vi "Actor Core.vi"(8 "error in":errorcluster, 11 "Top Level in":refnum<class "Top Level.lvclass">) -> (0 "error out":errorcluster, 3 "Actor out":refnum<class "Actor.lvclass">)   [LabVIEW 2020, in "2. Basic Panel Actors.lvlib" / "Top Level.lvclass"]
doc: "The user interface for this panel.\n----\nCopyright: MGI 2016\nAuthor: Derek Trepanier"
uses:
  Top Level.lvclass
  C:/Program Files/National Instruments/LabVIEW 2020/vi.lib/MGI/Panel Manager/Panel Actor/Panel Actor/Panel Actor.lvclass
  <vilib>/ActorFramework/Actor/Actor.lvclass
  <vilib>/ActorFramework/Message Enqueuer/Message Enqueuer.lvclass/Message Enqueuer.ctl
  Instrument/DMM/DMM.lvclass
  Instrument/Power Supply/Power Supply.lvclass
  <vilib>/ActorFramework/Message Enqueuer/Enqueue.vi
  Description Panel/Description Panel.lvclass
  <vilib>/MGI/Panel Manager/Panel/Panel/Subpanel/Subpanel.lvclass
  C:/Program Files/National Instruments/LabVIEW 2020/vi.lib/MGI/Panel Manager/Panel/Panel/Panel.lvclass
  <vilib>/ActorFramework/Stop Msg/Stop Msg.lvclass
  C:/Program Files/National Instruments/LabVIEW 2020/vi.lib/ActorFramework/Message/Message.lvclass
  <vilib>/MGI/Panel Manager/Panel/Panel/Window/Window.lvclass
  <vilib>/MGI/Panel Manager/Panel/Panel/Subpanel/Subpanel.vi
  <vilib>/ActorFramework/Message Priority Queue/Priority Enqueue.vi
  <vilib>/MGI/Panel Manager/Panel/Panel/Window/Window.vi
  <vilib>/MGI/Panel Manager/Panel Actor/Panel Actor/Panel Actor.lvclass
  <vilib>/MGI/Panel Manager/Panel/Panel.lvlib
panel:
  in  "Config Power Supply":bool
  in  "Config DMM":bool
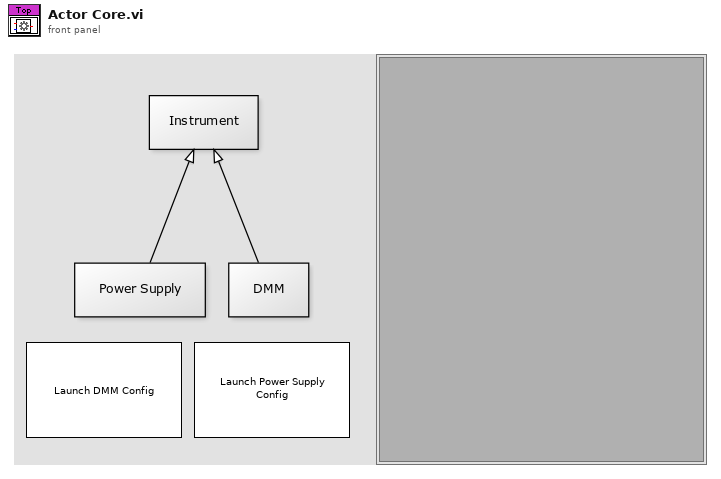
[diagram p1: front panel]
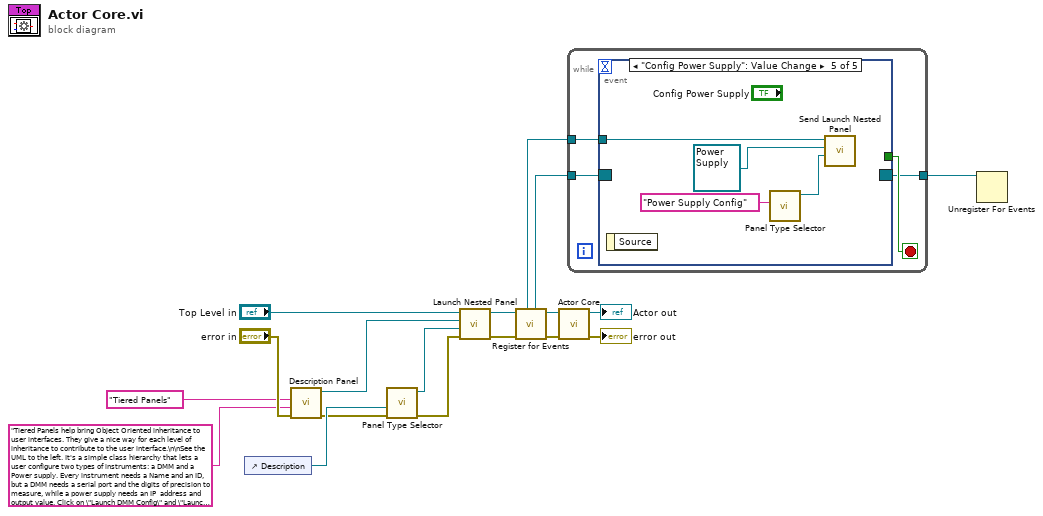
[diagram p0: block diagram]
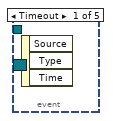
[diagram p2: hidden frame]
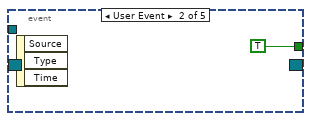
[diagram p3: hidden frame]
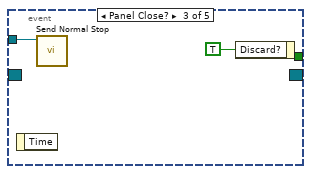
[diagram p4: hidden frame]
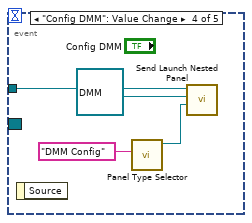
[diagram p5: hidden frame]
diagram:
  n1 = control-ref of="Description"() -> (w8:refnum<vi>)
  n2 = call "Description Panel.vi"("error in (no error)"="error in", "Description"="Tiered Panels help bring Object Oriented inheritance to user interfaces. They give a nice way for each level of inheritance to contribute to the user interface.\n\nSee the UML to the left. It's a simple class hierarchy that lets a user configure two types of instruments: a DMM and a Power supply. Every instrument needs a Name and an ID, but a DMM needs a serial port and the digits of precision to measure, while a power supply needs an IP  address and output value. Click on \"Launch DMM Config\" and \"Launch Power Supply Config\" and compare the two user interfaces. They both have the same \"Name\", \"ID\", and \"Save\" controls, but they have different \"Configuration\" controls.\n\nNow look at the Power Supply Config user interface. It's the Front Panel of \"Power Supply.lvclass:Actor Core.vi\". Notice how it only has the power supply specific controls. Just like how \"DMM.lvclass:Actor Core.vi\" only contains the DMM Specific controls.\n\nFinally, look at the Insturment's user interface in \"Instrument.lvclass:Actor Core.vi\". This contains only controls that are specific to <b>all</b> instruments, like the Name and the ID, as well as a button to save the configuration. It also contains a subpanel. This is where the specific instrument's UI will be inserted. Check out the block diagram of the Instrument's UI to see how to implement this. The bookmark <b>#TieredPanels</b> will explain how to make this work.\n" ("Description Title"), "Description Title"="Tiered Panels") -> ("error out"=w7:errorcluster, "Description Panel out"=w6:refnum<class "Description Panel.lvclass">)  [unwired: 7 in]
  n3 = call-poly <vilib>:"Panel Type Selector.vi"("Error In"=w7, "Sub Panel"=w8) -> ("Error Out"=w9:errorcluster, "Subpanel Out"=w2:refnum<class "Subpanel.lvclass">)  [unwired: 8 in]
  n4 = call <vilib>:"Launch Nested Panel.vi"("error in (no error)"=w9, "Panel"=w2, "Nested Panel Actor"=w6, "Panel Actor in"="Top Level in") -> ("error out"=w12:errorcluster, "Panel Actor out"=w10:refnum<class "Top Level.lvclass">)  [unwired: 4 in, 2 out]
  n5 = call <vilib>:"Register for Events.vi"("Error In"=w12, "Panel Actor in"=w10) -> ("Error Out"=w16:errorcluster, "Panel Actor out"=w15:refnum<class "Top Level.lvclass">, "Pnl Actor"=w14:refnum<event-registration>, "Self Enqueuer"=w13:refnum<class "Message Enqueuer.lvclass">)  [unwired: 6 in]
  n6 = call-parent "Actor Core.vi"("error in"=w16, "Panel Actor in"=w15) -> ("error out"=→"error out":errorcluster, "Actor out"=→"Actor out":refnum<class "Actor.lvclass">)  [unwired: 8 in]
  n7 = while {
    tunnel: w14 -> [w22]
    tunnel: w13 -> [w20]
    tunnel: [w19] -> w1
    stop <- w21 stop-if-true
    n8 = event shown="[4] \"Config Power Supply\": Value Change" {
      selector: w22 -> [_ _ _ _ _]
      dyn-events: [_ _ _ _ _] -> w19
      timeout: _ -> [_ _ _ _ _]
      tunnel: [_ TRUE _ _ _] -> w21
      tunnel: w20 -> [_ _ w24 w29 w33]
      event Timeout {
        n9 = event-data() -> ()  [unwired: 1 in, 3 out]
      }
      event User Event {
        n10 = event-data() -> ()  [unwired: 1 in, 3 out]
      }
      event Panel Close? {
        n11 = event-data() -> ()  [unwired: 1 in, 1 out]
        n12 = call <vilib>:"Send Normal Stop.vi"("Message Enqueuer"=w24) -> ()  [unwired: 10 in, 1 out]
        n13 = event-data("Discard?"=TRUE) -> ()  [unwired: 1 in, 1 out]
      }
      event "Config DMM": Value Change {
        n14 = event-data() -> ()  [unwired: 1 in, 1 out]
        n15 = call-poly <vilib>:"Panel Type Selector.vi"("Default Title"="DMM Config") -> ("Window out"=w27:refnum<class "Window.lvclass">)  [unwired: 9 in, 1 out]
        n16 = call <vilib>:"Send Launch Nested Panel.vi"("Panel"=w27, "Nested Panel Actor"=refnum<class "DMM.lvclass"> refnum ("2. Basic Panel Actors.lvlib:DMM.lvclass"), "Self Enqueuer in"=w29) -> ()  [unwired: 7 in, 2 out]
      }
      event "Config Power Supply": Value Change {
        n17 = event-data() -> ()  [unwired: 1 in, 1 out]
        n18 = call-poly <vilib>:"Panel Type Selector.vi"("Default Title"="Power Supply Config") -> ("Window out"=w32:refnum<class "Window.lvclass">)  [unwired: 9 in, 1 out]
        n19 = call <vilib>:"Send Launch Nested Panel.vi"("Panel"=w32, "Nested Panel Actor"=refnum<class "Power Supply.lvclass"> refnum ("2. Basic Panel Actors.lvlib:Power Supply.lvclass"), "Self Enqueuer in"=w33) -> ()  [unwired: 7 in, 2 out]
      }
    }
  }
  n20 = Unregister For Events(event registration refnum=w1) -> ()  [unwired: 1 in, 1 out]
